vi "Sort Auto Sequence Data's.vi"(8 "error in (no error)":errorcluster, 11 "Table":T2(array[cluster])) -> (0 "error out":errorcluster, 3 "Sorted AS Data":T1(array[cluster]))   [LabVIEW 2021, in "Test Configuration.lvlib"]
uses:
  Test Configuration.lvlib
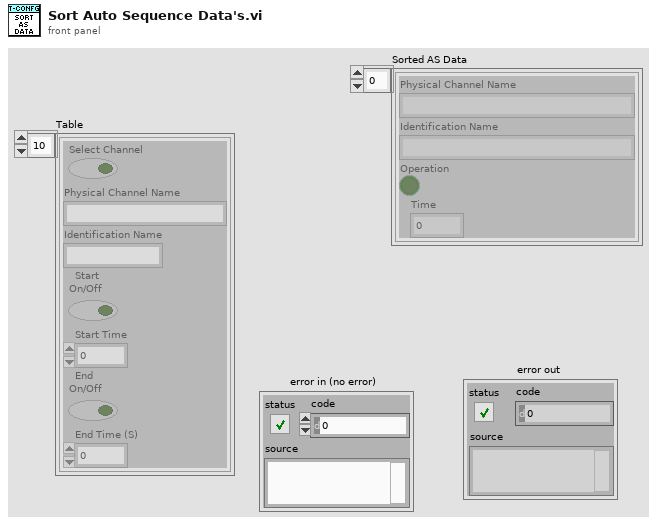
[diagram p1: front panel]
types:
  T1 = cluster{"Physical Channel Name":string, "Identification Name":string, "Operation":bool, "Time":dbl}[]
  T2 = cluster{"Select Channel":bool, "Physical Channel Name":string, "Identification Name":string, "  Start\nOn/Off":bool, "Start Time":dbl, "  End\nOn/Off":bool, "End Time (S)":dbl}[]
  T3 = cluster{"Physical Channel Name":string, "Channel Name":string, "Operation":bool, "Time":dbl}
  T4 = cluster{"Physical Channel Name":string, "Identification Name":string, "Operation":bool, "Time":dbl}
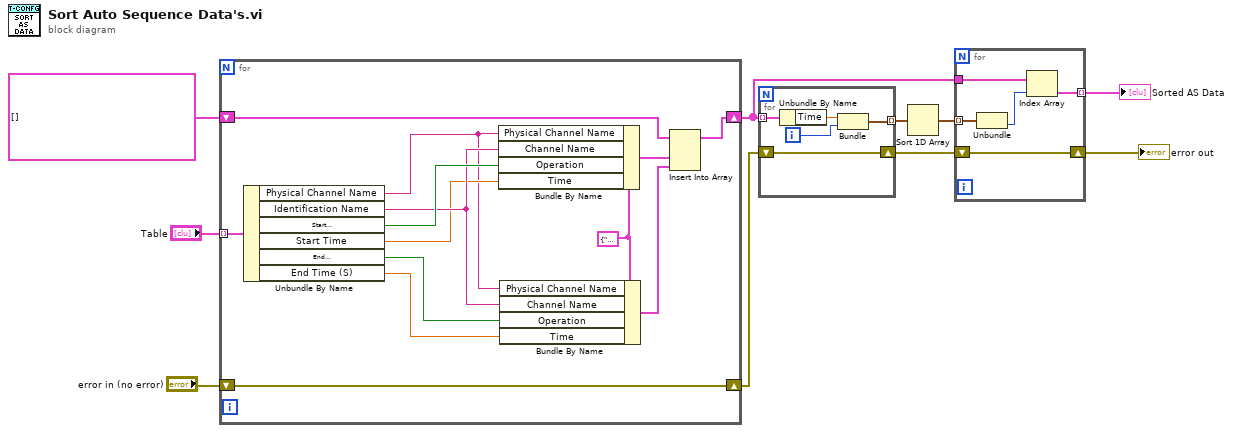
[diagram p0: block diagram]
diagram:
  n1 = for {
    tunnel: "Table" -> [w23] mode=indexing
    shift-right: [w17] -> w8
    shift-left: T1 [] -> [w19]
    shift-right: [w11] -> w4
    shift-left: "error in (no error)" -> [w11]
    w15 = T3 {"Physical Channel Name"="", "Channel Name"="", "Operation"=FALSE, "Time"=0.0} ("Cluster")
    n2 = Unbundle By Name(w23) -> ("Physical Channel Name"=w12:string, "Identification Name"=w21:string, "Start\nOn/Off"=w22:bool, "Start Time"=w16:dbl, "End\nOn/Off"=w20:bool, "End Time (S)"=w18:dbl)
    n3 = Bundle By Name(cluster=w15, "Physical Channel Name"=w12, "Channel Name"=w21, "Operation"=w22, "Time"=w16) -> (w14:T3)
    n4 = Bundle By Name(cluster=w15, "Physical Channel Name"=w12, "Channel Name"=w21, "Operation"=w20, "Time"=w18) -> (w13:T3)
    n5 = Insert Into Array(array=w19, new element #1=w14, new element #2=w13) -> (w17:T1)  [unwired: 1 in]
  }
  n6 = for {
    tunnel: w8 -> [w28] mode=indexing
    tunnel: [w27] -> w10 mode=indexing
    shift-right: [w24] -> w3
    shift-left: w4 -> [w24]
    i -> [w25]
    n7 = Unbundle By Name(w28) -> ("Time"=w26:dbl)
    n8 = Bundle("Time"=w26, w25) -> (w27:cluster{"Time":dbl, i32})  [unwired: 1 in]
  }
  n9 = Sort 1D Array(array=w10) -> (sorted array=w9:cluster{"Time":dbl, i32}[])
  n10 = for {
    tunnel: w9 -> [w33] mode=indexing
    tunnel: w8 -> [w32]
    tunnel: [w31] -> w1 mode=indexing
    shift-right: [w29] -> w2
    shift-left: w3 -> [w29]
    n11 = Unbundle(w33) -> (w30:i32)  [unwired: 1 out]
    n12 = Index Array(array=w32, index=w30) -> (element=w31:T4)
  }
  "error out" <- w2
  "Sorted AS Data" <- w1
